vi "CloseConnectionInternal.vi"(8 "error in (no error)":errorcluster, 9 "Qbus in":refnum<class "Qbus.lvclass">, 10 "connected":T2, 11 "tcp":T1) -> (0 "error out":errorcluster)   [LabVIEW 2017, in "ServerComm.lvlib"]
uses:
  <vilib>/addons/InsightCM/Devices/Shared/Common/ServerComm/ServerComm.lvlib
  <vilib>/addons/InsightCM/Devices/Shared/Common/ServerComm/controls/ConnectedStatusDvr.ctl
  <vilib>/addons/InsightCM/Devices/Shared/Common/ServerComm/controls/ConnectionStatus.ctl
  <vilib>/addons/InsightCM/MessageBus/TcpApi/controls/TcpMessageReference.ctl
  <vilib>/addons/Qbus/Qbus.lvclass
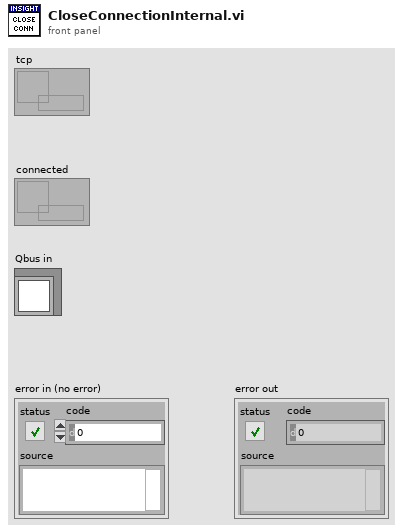
[diagram p1: front panel]
types:
  T1 = typedef "TcpMessageReference.ctl" = refnum<data-value>
  T2 = typedef "ServerComm.lvlib/ConnectedStatusDvr.ctl" = refnum<data-value>
  T3 = typedef "ServerComm.lvlib/ConnectionStatus.ctl" = enum16{"Offline", "NotAuthorized", "Online"}
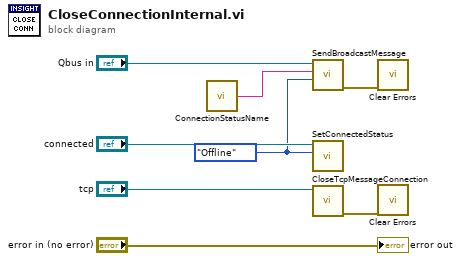
[diagram p0: block diagram]
diagram:
  w3 = ConnectionStatus."Offline" ("status")
  n1 = call <vilib>:"ConnectionStatusName.vi"() -> ("message name"=w1:string)  [unwired: 5 in]
  n2 = call <vilib>:"SendBroadcastMessage.vi"("message value"=w3, "message name"=w1, "Qbus in"="Qbus in") -> ("error in (no error)"=w2:errorcluster)  [unwired: 7 in, 1 out]
  n3 = call <vilib>:"SetConnectedStatus.vi"("status"=w3, "dvrConnected"="connected") -> ()  [unwired: 5 in, 1 out]
  n4 = call <vilib>:"CloseTcpMessageConnection.vi"("connection ID in"="tcp") -> ("error out"=w5:errorcluster)  [unwired: 10 in]
  n5 = call <vilib>:"Clear Errors.vi"("error in (no error)"=w2) -> ()  [unwired: 5 in, 2 out]
  n6 = call <vilib>:"Clear Errors.vi"("error in (no error)"=w5) -> ()  [unwired: 5 in, 2 out]
  "error out" <- "error in (no error)"
